vi "DeadBand.vi"(8 "Deadband":dbl, 11 "Input":dbl) -> (3 "Output":dbl)   [LabVIEW 2018]
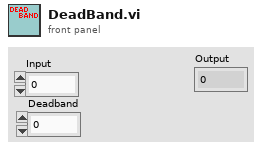
[diagram p1: front panel]
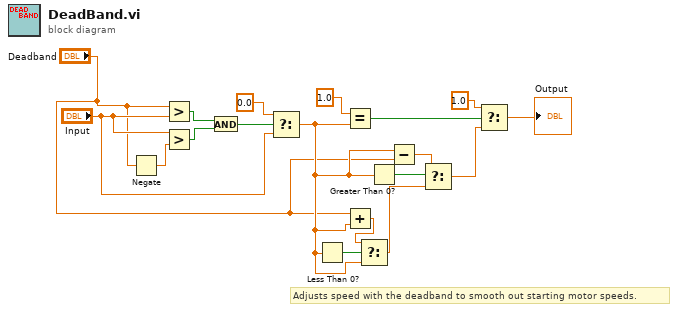
[diagram p0: block diagram]
diagram:
  # "Adjusts speed with the deadband to smooth out starting motor speeds."
  n1 = Negate(x="Deadband") -> (-x=w13:dbl)
  n2 = Greater?(x="Deadband", y="Input") -> (0:w18:bool)
  n3 = Greater?(x="Input", y=w13) -> (0:w17:bool)
  n4 = And(x=w18, y=w17) -> (x .and. y?=w16:bool)
  n5 = Select(t=0.0, s=w16, f="Input") -> (s? t:f=w2:dbl)
  n6 = Less Than 0?(x=w2) -> (x < 0?=w5:bool)
  n7 = Equal?(x=1.0, y=w2) -> (x = y?=w11:bool)
  n8 = Add(x="Deadband", y=w2) -> (x+y=w4:dbl)
  n9 = Select(t=w4, s=w5, f=w2) -> (s? t:f=w6:dbl)
  n10 = Greater Than 0?(x=w2) -> (x > 0?=w7:bool)
  n11 = Subtract(x=w2, y="Deadband") -> (x-y=w8:dbl)
  n12 = Select(t=w8, s=w7, f=w6) -> (s? t:f=w3:dbl)
  n13 = Select(t=1.0, s=w11, f=w3) -> (s? t:f=→"Output":dbl)
